vi "Pre Launch Init.vi"(11 "Single Assert Display in":refnum<class "Single Assert Display.lvclass">) -> (0 "error out":errorcluster, 3 "Single Assert Display out":refnum<class "Single Assert Display.lvclass">)   [LabVIEW 2016, in "Assert API Components.lvlib" / "Assert Display.lvlib" / "Single Assert Display.lvlib" / "Single Assert Display.lvclass"]
doc: "(<B>Filename</B>: Actor Framework.lvlib:Actor.lvclass:Pre Launch Init.vi)\n\nDefines behavior that occurs after the Launch Nested Actor method is invoked but before the actor's Actor Core method begins running.\n\nBy default, this method does nothing. A descendant class may override it to define behavior."
uses:
  Single Assert Display.lvclass
  Assert API Components/Message Data.ctl
  Assert API Components/VI References.ctl
  Single Assert Display.lvclass/Single Assert Display.ctl
  Base UI Actor/Base UI Actor/Base UI Actor.lvclass
  Assert API Components/Assert API Components.lvlib
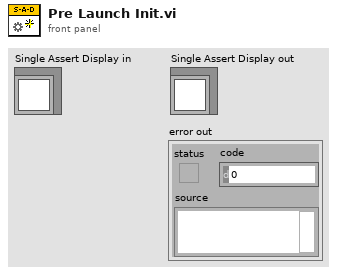
[diagram p1: front panel]
types:
  T1 = typedef "Assert API Components.lvlib/Message Data.ctl" = cluster{"Data Value":variant, "Last Update":timestamp, "Comment":string, "Evaluation String":string, "Status":bool, "Assert Name":string, "Failure Action":string, "Assert VI Name":string, "Calling VI Name":string, "Assert VI UID":i32, "Top Level VI Name":string, "VI References":T2, "Assert Build Timestamp":timestamp, "Assert Builder User Name":string, "Data Type":string}
  T2 = typedef "Assert API Components.lvlib/VI References.ctl" = cluster{"Calling VI Ref":refnum<vi>, "Assert VI Ref":refnum<vi>}
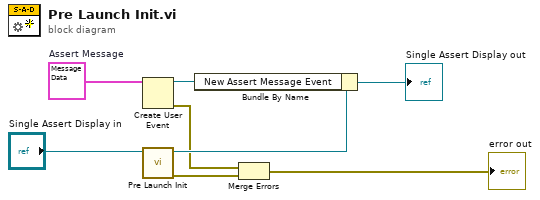
[diagram p0: block diagram]
diagram:
  w5 = T1 {"Data Value"=variant, "Last Update"=timestamp(0 s since 1904-01-01), "Comment"="", "Evaluation String"="", "Status"=FALSE, "Assert Name"="", "Failure Action"="", "Assert VI Name"="", "Calling VI Name"="", "Assert VI UID"=0, "Top Level VI Name"="", "VI References"={"Calling VI Ref"=refnum, "Assert VI Ref"=refnum}, "Assert Build Timestamp"=timestamp(0 s since 1904-01-01), "Assert Builder User Name"="", "Data Type"=""}  # Assert Message
  n1 = Create User Event(user event datatype=w5) -> (user event=w3:refnum<user-event>, error out=w1:errorcluster)  [unwired: 1 in]
  n2 = call-parent "Pre Launch Init.vi"("Base UI Actor in"="Single Assert Display in") -> ("error out"=w8:errorcluster, "Base UI Actor out"=w7:refnum<class "Single Assert Display.lvclass">)  [unwired: 9 in]
  n3 = Bundle By Name(cluster=w7, "New Assert Message Event"=w3) -> (→"Single Assert Display out":refnum<class "Single Assert Display.lvclass">)
  n4 = Merge Errors(w1, w8) -> (→"error out":errorcluster)
